vi "IMAQdx Serial Flush.vi"(8 "error in":errorcluster, 11 "Session In":T1) -> (0 "error out":errorcluster, 3 "Session Out":T1)   [LabVIEW 2020, in "NI_Vision_Acquisition_Software.lvlib"]
doc: "Flushes data from the serial port read buffer on image acquisition devices that support serial communication."
uses:
  NI_Vision_Acquisition_Software.lvlib
  IMAQdx.ctl
  niimaqdx.dll
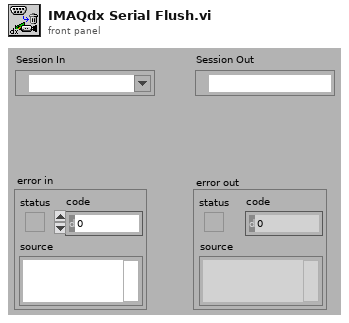
[diagram p1: front panel]
types:
  T1 = typedef "IMAQdx.ctl" = refnum<k21>
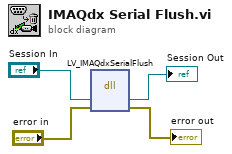
[diagram p0: block diagram]
diagram:
  n1 = dll-call lib="niimaqdx.dll" fn="LV_IMAQdxSerialFlush"("refnum"="Session In", "error"="error in") -> ("refnum"=→"Session Out":T1, "error"=→"error out":errorcluster)  [unwired: 4 in, 2 out]
